vi "XNET Bus Monitor Main Service.vi"(10 "Global Stop":refnum<notifier>, 11 "Name in":string="CANBusMonitor") -> ()   [LabVIEW 2025]
uses:
  Support Code/XNET.CAN.BusMonitor.API.lvclass
panel:
  out "IP":string="localhost"
  out "Name":string="CANBusMonitor"
  out "Listening Port":i32
  out "gRPC Server Status":string
  out "gRPC error out":errorcluster
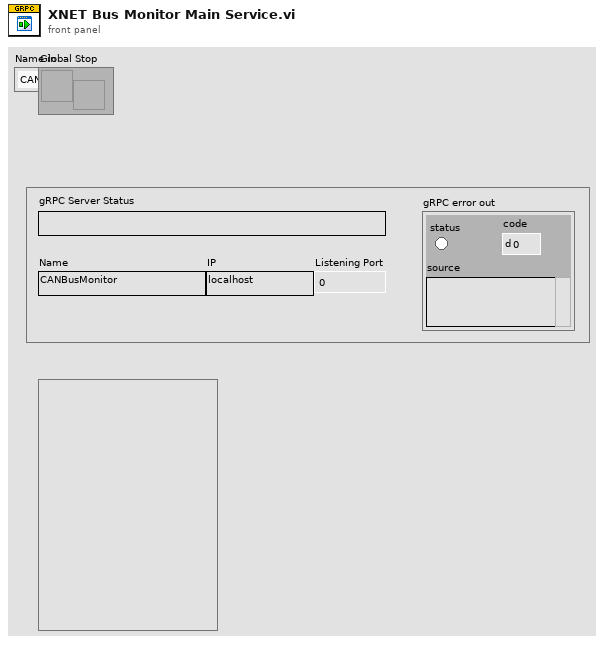
[diagram p1: front panel]
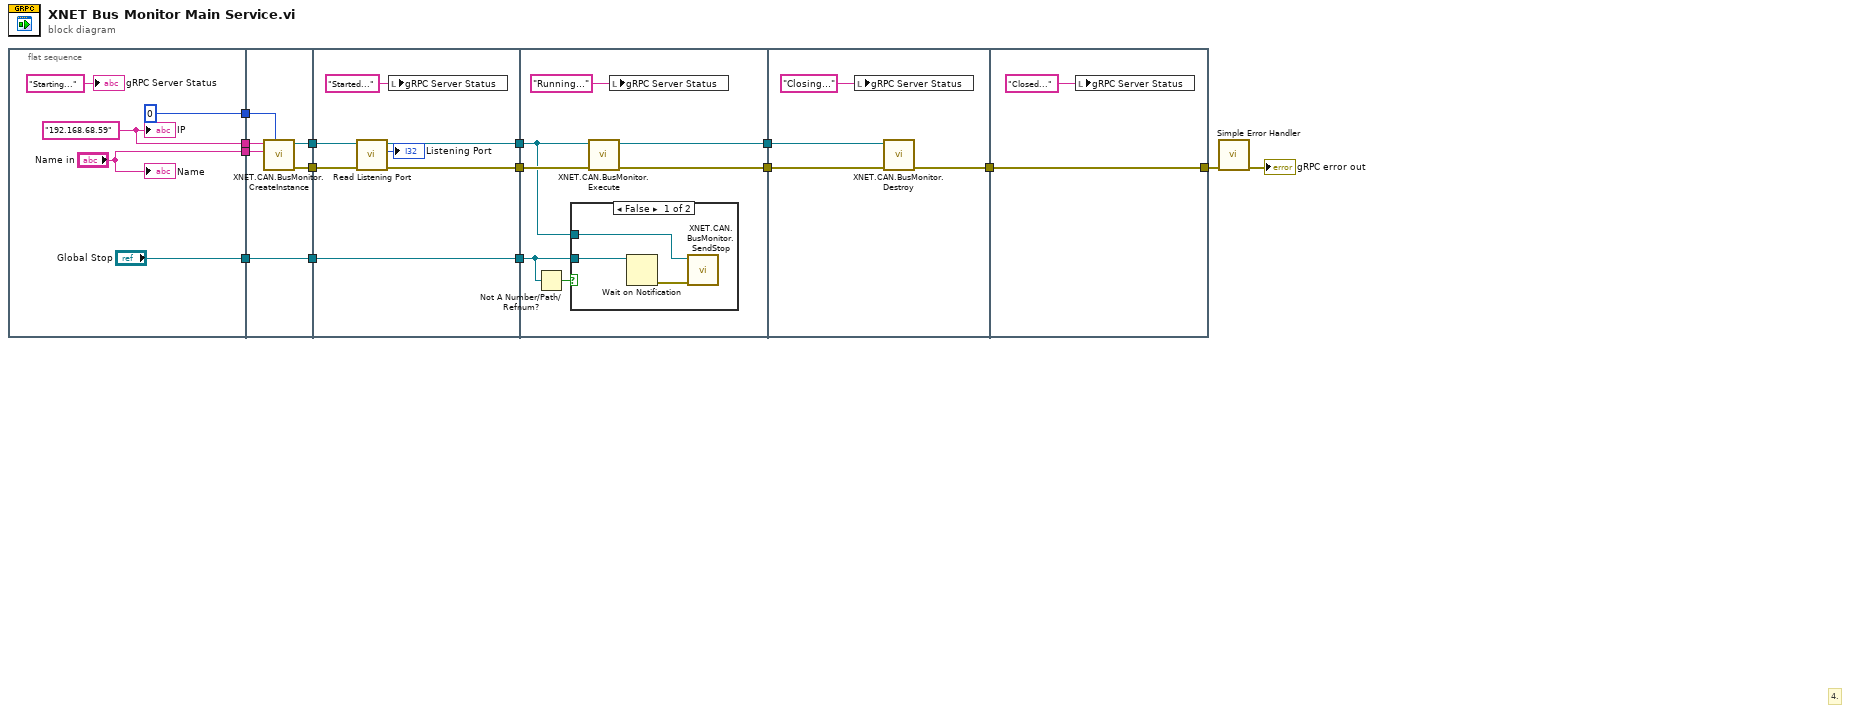
[diagram p0: block diagram]
diagram:
  # "4."
  n1 = flat-sequence {
    tunnel: [w20] -> w14
    tunnel: ["Name in"] -> w13
    tunnel: [0 ("Listening Port (0 = auto)")] -> w12
    tunnel: ["Global Stop"] -> w1
    tunnel: w14 -> [w24]
    tunnel: w13 -> [w25]
    tunnel: w12 -> [w26]
    tunnel: [w23] -> w11
    tunnel: [w22] -> w10
    tunnel: [w21] -> w2
    tunnel: w1 -> [w21]
    tunnel: w11 -> [w32]
    tunnel: w10 -> [w28]
    tunnel: [w31] -> w9
    tunnel: [w30] -> w8
    tunnel: [w27] -> w3
    tunnel: w2 -> [w27]
    tunnel: w9 -> [w40]
    tunnel: w8 -> [w34]
    tunnel: [w39] -> w7
    tunnel: [w38] -> w6
    tunnel: w3 -> [w35]
    tunnel: w7 -> [w46]
    tunnel: w6 -> [w45]
    tunnel: [w44] -> w4
    tunnel: [w49] -> w5
    tunnel: w4 -> [w49]
    frame #0 {
      w20 = "192.168.68.59" ("IP")
      "gRPC Server Status" <- "Starting..." ("String")
      "Name" <- "Name in"
      "IP" <- w20
    }
    frame #1 {
      n2 = call "XNET.CAN.BusMonitor.CreateInstance.vi"("Listening Port (0 = auto)"=w26, "Name"=w25, "IP"=w24) -> ("error out"=w23:errorcluster, "gRPC Container out"=w22:refnum<class "XNET.CAN.BusMonitor.API.lvclass">)  [unwired: 7 in]
    }
    frame #2 {
      n3 = call-dynamic "Read Listening Port.vi"("error in (no error)"=w32, "gRPC Container in"=w28) -> ("error out"=w31:errorcluster, "Listening Port"=→"Listening Port":i32, "gRPC Container out"=w30:refnum<class "XNET.CAN.BusMonitor.API.lvclass">)  [unwired: 7 in]
      n4 = local write "gRPC Server Status"("Started..." ("gRPC Server Status")) -> ()
    }
    frame #3 {
      n5 = Not A Number/Path/Refnum?(number/path/refnum=w35) -> (NaN/Path/Refnum?=w36:bool)
      n6 = case shown="False" w36 {
        tunnel: w35 -> [w42 _]
        tunnel: w34 -> [w41 _]
        frame False {
          n7 = Wait on Notification(notifier=w42) -> (error out=w43:errorcluster)  [unwired: 3 in, 3 out]
          n8 = call-dynamic "XNET.CAN.BusMonitor.SendStop.vi"("error in (no error)"=w43, "gRPC Container in"=w41) -> ()  [unwired: 8 in, 2 out]
        }
        frame True {
        }
      }
      n9 = call-dynamic "XNET.CAN.BusMonitor.Execute.vi"("error in (no error)"=w40, "gRPC Container in"=w34) -> ("error out"=w39:errorcluster, "gRPC Container out"=w38:refnum<class "XNET.CAN.BusMonitor.API.lvclass">)  [unwired: 8 in]
      n10 = local write "gRPC Server Status"("Running..." ("gRPC Server Status")) -> ()
    }
    frame #4 {
      n11 = local write "gRPC Server Status"("Closing..." ("gRPC Server Status")) -> ()
      n12 = call-dynamic "XNET.CAN.BusMonitor.Destroy.vi"("error in (no error)"=w46, "gRPC Container in"=w45) -> ("error out"=w44:errorcluster)  [unwired: 8 in, 1 out]
    }
    frame #5 {
      n13 = local write "gRPC Server Status"("Closed..." ("gRPC Server Status")) -> ()
    }
  }
  n14 = call <vilib>:"Simple Error Handler.vi"("error in (no error)"=w5) -> ("error out"=→"gRPC error out":errorcluster)  [unwired: 1 in, 7 out]
